vi "SR830_Close.vi"(8 "Error In":errorcluster caption="错误输入", 11 "VISA 输入":refnum<visa-resource-name>="GPIB0::7::INSTR") -> (0 "Error Out":errorcluster caption="错误输出")   [LabVIEW 2020]
uses:
  lib/SR830/SR830.lvlib
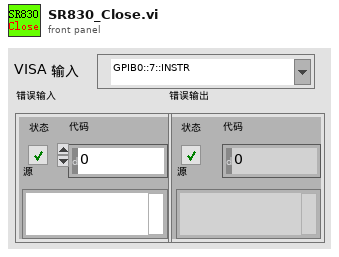
[diagram p1: front panel]
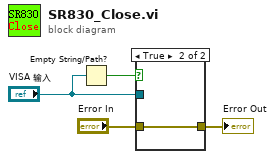
[diagram p0: block diagram]
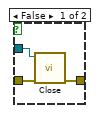
[diagram p2: hidden frame]
diagram:
  n1 = Empty String/Path?(string/path="VISA 输入") -> (empty?=w1:bool)
  n2 = case shown="True" w1 {
    tunnel: "Error In" -> [w7 w8]
    tunnel: "VISA 输入" -> [w6 _]
    tunnel: [w5 w8] -> w4
    frame False {
      n3 = call "Close.vi"("error in (no error)"=w7, "VISA resource name"=w6) -> ("error out"=w5:errorcluster)  [unwired: 9 in]
    }
    frame True {
    }
  }
  "Error Out" <- w4
